vi "Config Digital Output.vi"(0 "VISA resource name":refnum<visa-resource-name>, 5 "Digital Output\nMode (0: Off)":u16(ring) items=["Off", "Alarms", "Scanner", "Manual"], 7 "Manual Output\nValue (0)":dbl min=0.0 max=31.0 step=1.0, 11 "error in (no error)":errorcluster) -> (4 "VISA resource name out":refnum<visa-resource-name>, 15 "error out":errorcluster)   [LabVIEW 2024, in "Lake Shore Cryotronics 340.lvlib"]
doc: "This VI configures the parameters of the digital output."
uses:
  Lake Shore Cryotronics 340.lvlib
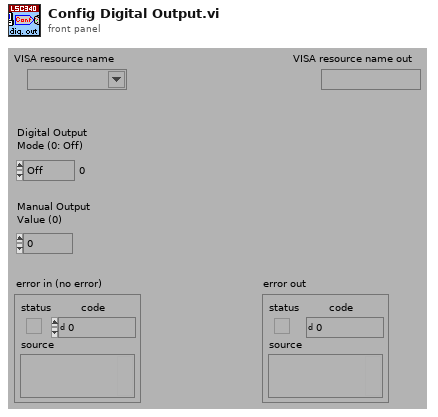
[diagram p1: front panel]
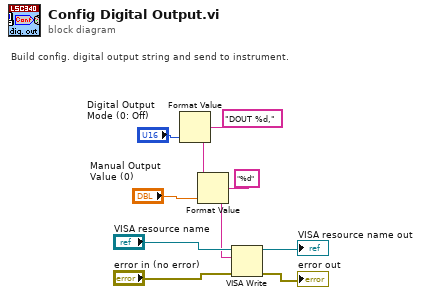
[diagram p0: block diagram]
diagram:
  # "Build config. digital output string and send to instrument."
  n1 = Format Value(format string="DOUT %d,", value (0)="Digital Output\nMode (0: Off)") -> (output string=w7:string)  [unwired: 1 in]
  n2 = Format Value(string ("")=w7, format string="%d", value (0)="Manual Output\nValue (0)") -> (output string=w1:string)
  n3 = VISA Write(VISA resource name="VISA resource name", write buffer=w1, error in (no error)="error in (no error)") -> (VISA resource name out=→"VISA resource name out":refnum<visa-resource-name>, error out=→"error out":errorcluster)  [unwired: 1 out]
